vi "getObject.vi"(1 "arrowHead":T1, 5 "error in (no error)":errorcluster) -> (14 "reference out":refnum<class "ArrowHead.lvclass">, 19 "error out":errorcluster)   [LabVIEW 2016, in "ArrowHead.lvclass"]
doc: "Gets an object"
uses:
  <resource>/Framework/Providers/Open_GDS/UML/ArrowHead_class/ArrowHead.lvclass
  <resource>/Framework/Providers/Open_GDS/UML/ArrowHead_class/ArrowHeadType.ctl
  <resource>/Framework/Providers/Open_GDS/UML/ArrowHead_class/ArrowHead.lvclass/ArrowHead.ctl
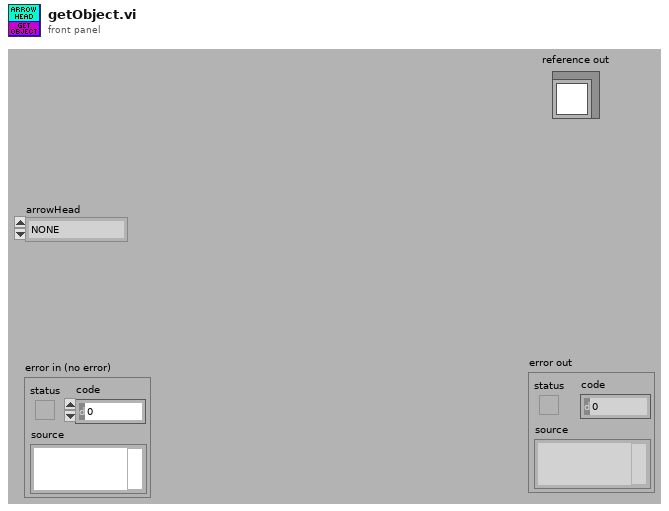
[diagram p1: front panel]
types:
  T1 = typedef "ArrowHead.lvclass/ArrowHeadType.ctl" = enum16{"NONE", "TRIANGLE", "BLACK_TRIANGLE", "V", "HALF_V", "DIAMOND", "BLACK_DIAMOND"}
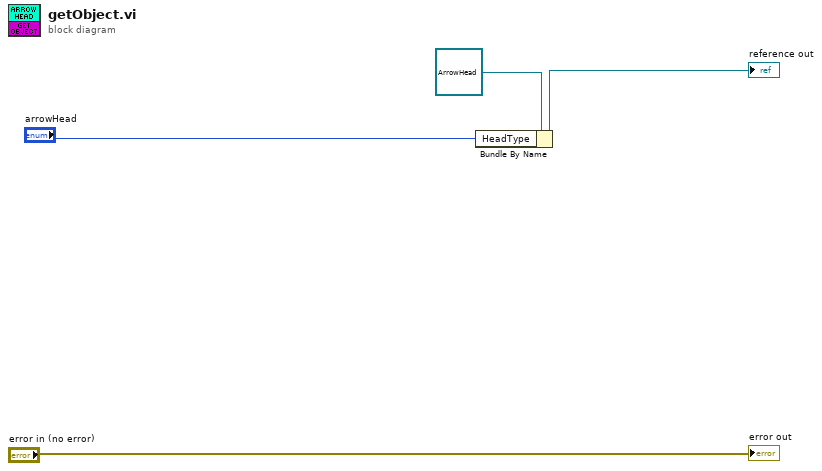
[diagram p0: block diagram]
diagram:
  n1 = Bundle By Name(cluster=refnum<class "ArrowHead.lvclass"> refnum ("NONE"), "HeadType"="arrowHead") -> (→"reference out":refnum<class "ArrowHead.lvclass">)
  "error out" <- "error in (no error)"
